vi "calculate 3d euclidean distance.vi"(0 "x1":dbl, 1 "y1":dbl, 2 "z1":dbl, 3 "x2":dbl, 4 "y2":dbl, 5 "z2":dbl) -> (14 "euclid dist":dbl)   [LabVIEW 2012]
doc: "SciScan 1.2 160622"
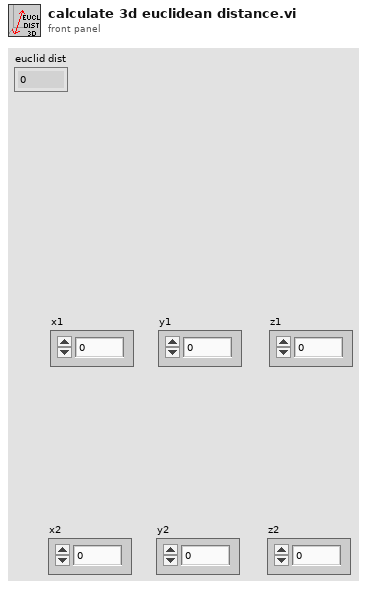
[diagram p1: front panel]
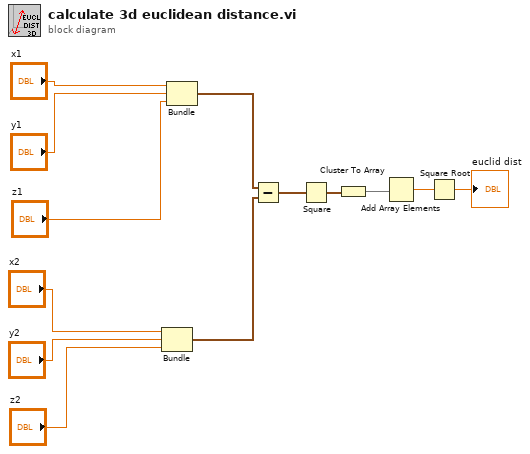
[diagram p0: block diagram]
diagram:
  n1 = Bundle("x2"="x2", "y2"="y2", "z2"="z2") -> (w6:cluster{"x2":dbl, "y2":dbl, "z2":dbl})  [unwired: 1 in]
  n2 = Bundle("x1"="x1", "y1"="y1", "z1"="z1") -> (w7:cluster{"x1":dbl, "y1":dbl, "z1":dbl})  [unwired: 1 in]
  n3 = Subtract(x=w7, y=w6) -> (x-y=w5:cluster{dbl, dbl, dbl})
  n4 = Square(x=w5) -> (x^2=w4:cluster{dbl, dbl, dbl})
  n5 = Cluster To Array(cluster=w4) -> (array=w3:dbl[])
  n6 = Add Array Elements(numeric array=w3) -> (sum=w2:dbl)
  n7 = Square Root(x=w2) -> (sqrt(x)=→"euclid dist":dbl)
